vi "APC_9049_FPGA_IGNDI_supervisor.vi"(1 "Time out limit":u32=6000000, 2 "EPTData":T1={"CrankSigOS"=FALSE, "CrankStalled"=FALSE, "SyncStopped"=FALSE, "MissedCrankFlag"=FALSE, "MissedCamFlag"=FALSE, "Period"=588, "PeriodAccum"=3882066, "CrankCount"=5844, "CurrentPosition"=23376, "MAX_CAT"=57600}, 3 "SIarray":bool[](array[boolean])=[FALSE, FALSE, FALSE, FALSE, FALSE, FALSE], 4 "DIarray":bool[](array[boolean])=[FALSE, FALSE, FALSE, FALSE, FALSE, FALSE]) -> (0 "NumberOfActiveIGN_DI":u8)   [LabVIEW 2020]
panel:
  out "Number of inactive injections":u8
  out "Number of inactive sparks":i16
  out "DI6":bool
  out "DI5":bool
  out "DI4":bool
  out "DI3":bool
  out "DI2":bool
  out "DI1":bool
  out "SI6":bool
  out "SI5":bool
  out "SI4":bool
  out "SI3":bool
  out "SI2":bool
  out "SI1":bool
  # "6e6 times out por 800 rpm\n\n2*60/rpm*40e10"
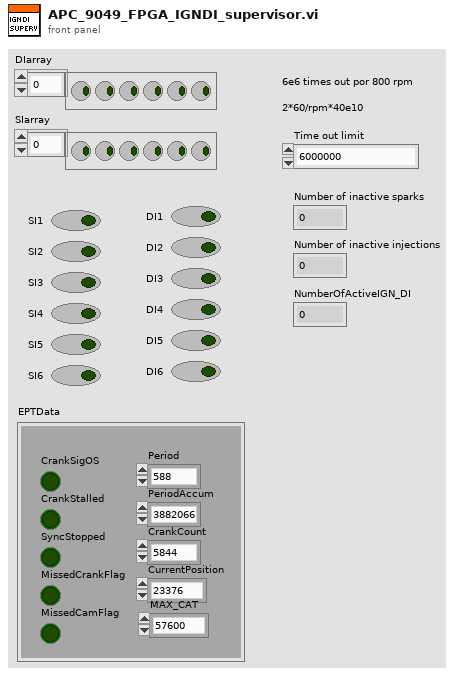
[diagram p1: front panel]
types:
  T1 = cluster{"CrankSigOS":bool, "CrankStalled":bool, "SyncStopped":bool, "MissedCrankFlag":bool, "MissedCamFlag":bool, "Period":u32, "PeriodAccum":u32, "CrankCount":u16, "CurrentPosition":u16, "MAX_CAT":u16}
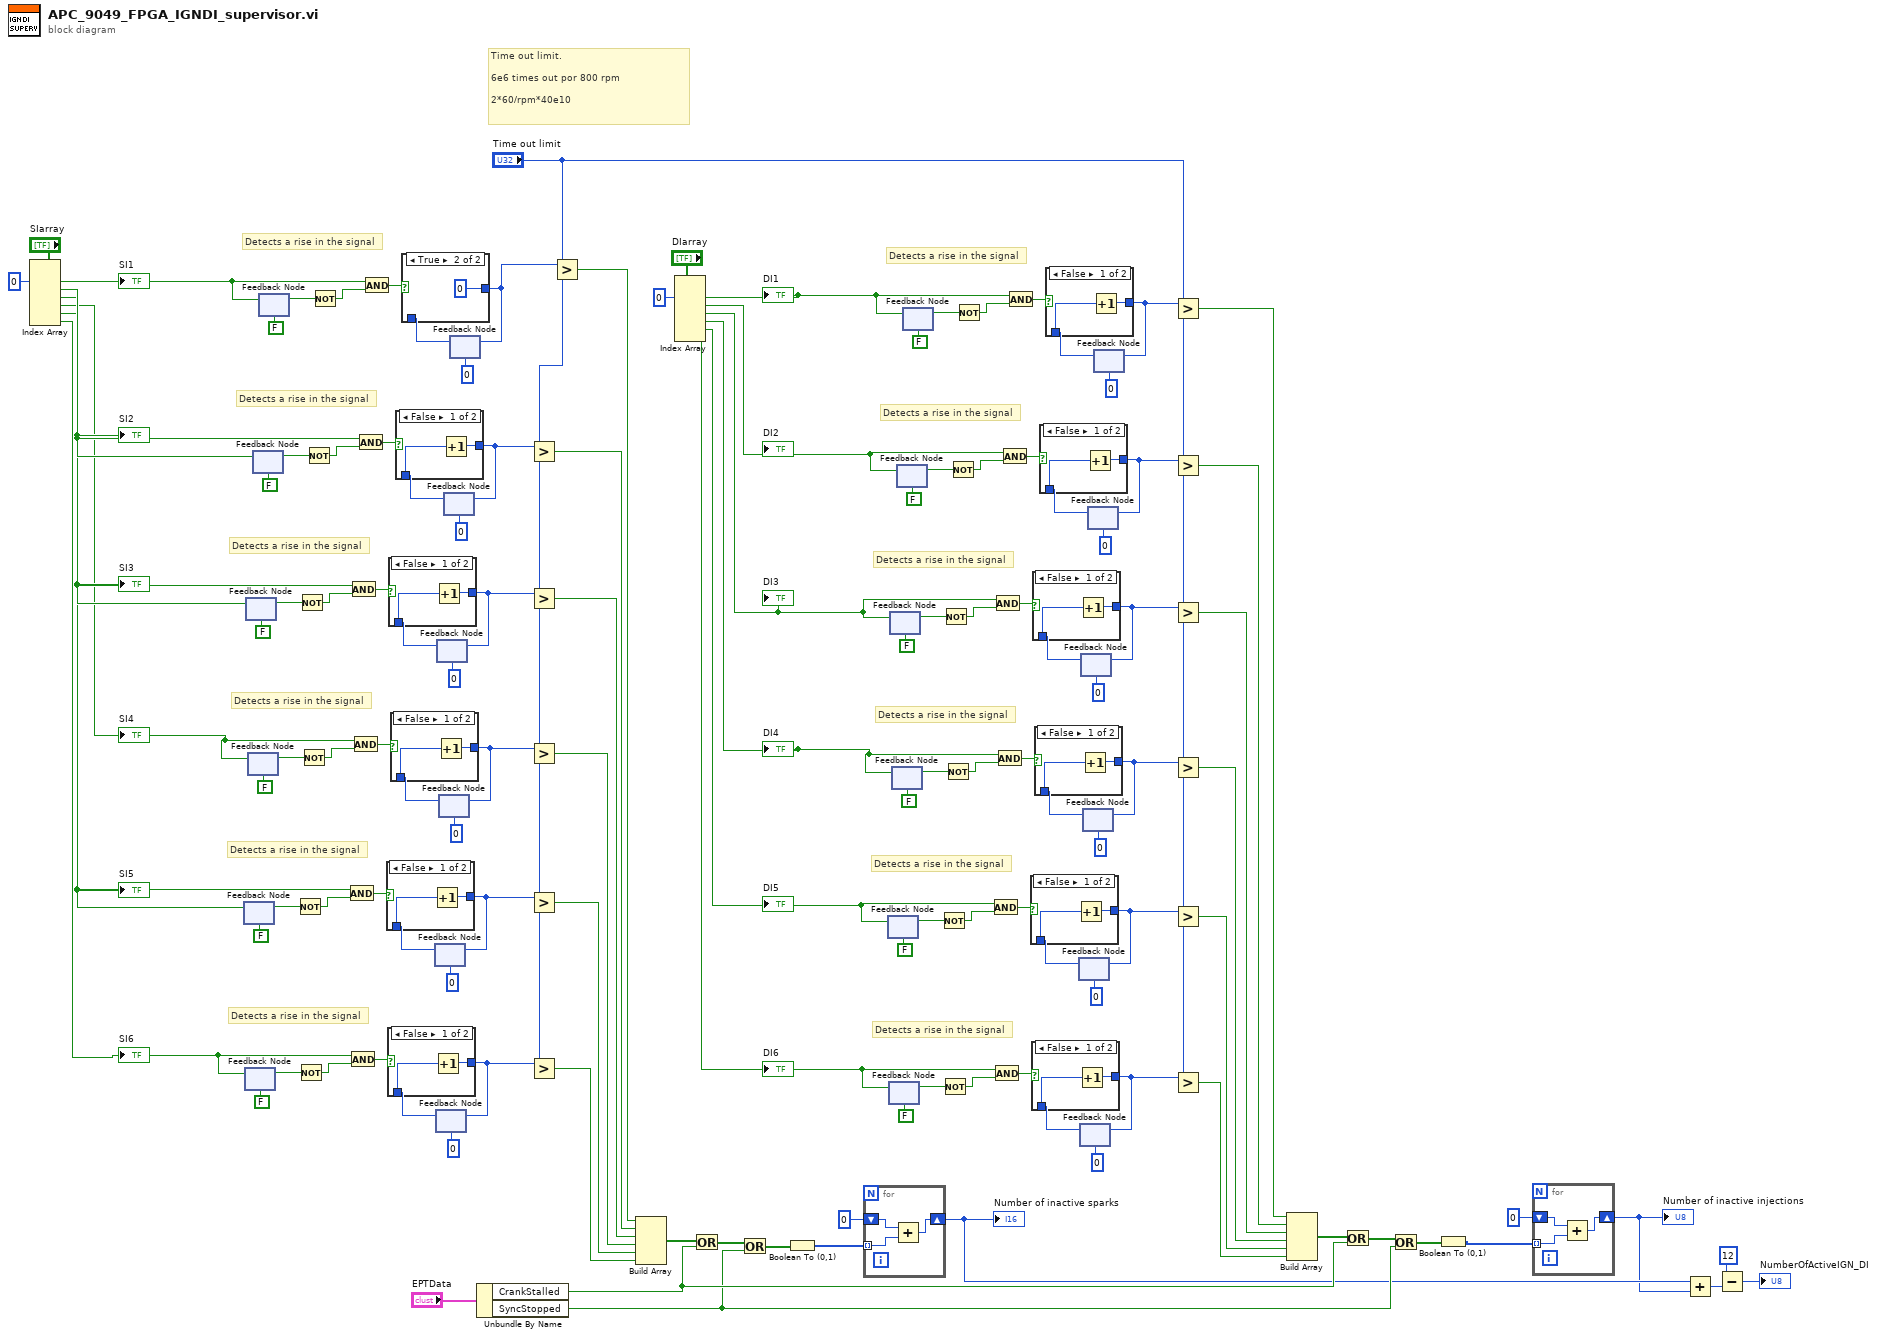
[diagram p0: block diagram]
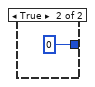
[diagram p2: hidden frame]
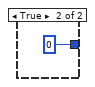
[diagram p3: hidden frame]
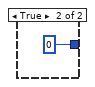
[diagram p4: hidden frame]
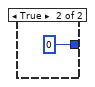
[diagram p5: hidden frame]
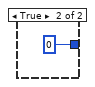
[diagram p6: hidden frame]
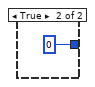
[diagram p7: hidden frame]
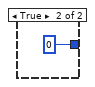
[diagram p8: hidden frame]
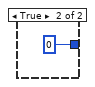
[diagram p9: hidden frame]
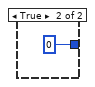
[diagram p10: hidden frame]
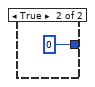
[diagram p11: hidden frame]
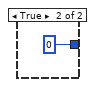
[diagram p12: hidden frame]
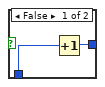
[diagram p13: hidden frame]
diagram:
  # "Detects a rise in the signal"
  # "Detects a rise in the signal"
  # "Detects a rise in the signal"
  # "Detects a rise in the signal"
  # "Detects a rise in the signal"
  # "Detects a rise in the signal"
  # "Detects a rise in the signal"
  # "Detects a rise in the signal"
  # "Detects a rise in the signal"
  # "Detects a rise in the signal"
  # "Detects a rise in the signal"
  # "Time out limit.\n\n6e6 times out por 800 rpm\n\n2*60/rpm*40e10"
  # "Detects a rise in the signal"
  n1 = Index Array(array="SIarray", index #1=0 ("index")) -> (element #1=w6:bool, element #2=w5:bool, element #3=w4:bool, element #4=w3:bool, element #5=w2:bool, element #6=w1:bool)  [unwired: 5 in]
  "SI1" <- w6
  "SI2" <- w5
  "SI3" <- w4
  "SI4" <- w3
  "SI5" <- w2
  "SI6" <- w1
  n2 = feedback #1(FALSE ("x")) -> (w101:bool)
  n3 = feedback-in #1(w2) -> ()
  n4 = feedback #2(FALSE ("x")) -> (w94:bool)
  n5 = feedback-in #2(w1) -> ()
  n6 = feedback #3(FALSE ("x")) -> (w115:bool)
  n7 = feedback-in #3(w4) -> ()
  n8 = feedback #4(FALSE ("x")) -> (w108:bool)
  n9 = feedback-in #4(w3) -> ()
  n10 = feedback #5(FALSE ("x")) -> (w122:bool)
  n11 = feedback-in #5(w5) -> ()
  n12 = feedback-in #6(w6) -> ()
  n13 = feedback #6(FALSE ("x")) -> (w130:bool)
  n14 = Not(x=w101) -> (.not. x?=w102:bool)
  n15 = Not(x=w94) -> (.not. x?=w95:bool)
  n16 = Not(x=w115) -> (.not. x?=w116:bool)
  n17 = Not(x=w108) -> (.not. x?=w109:bool)
  n18 = Not(x=w122) -> (.not. x?=w123:bool)
  n19 = Not(x=w130) -> (.not. x?=w131:bool)
  n20 = And(x=w2, y=w102) -> (x .and. y?=w99:bool)
  n21 = And(x=w1, y=w95) -> (x .and. y?=w92:bool)
  n22 = And(x=w4, y=w116) -> (x .and. y?=w113:bool)
  n23 = And(x=w3, y=w109) -> (x .and. y?=w106:bool)
  n24 = And(x=w5, y=w123) -> (x .and. y?=w120:bool)
  n25 = And(x=w6, y=w131) -> (x .and. y?=w128:bool)
  n26 = feedback #7(u32 0) -> (w98:u32)
  n27 = case shown="False" w99 {
    tunnel: [w133 u32 0] -> w96
    tunnel: w98 -> [w132 _]
    frame False {
      n28 = Increment(x=w132) -> (x+1=w133:u32)
    }
    frame True {
    }
  }
  n29 = feedback-in #7(w96) -> ()
  n30 = feedback #8(u32 0) -> (w91:u32)
  n31 = case shown="False" w92 {
    tunnel: [w136 u32 0] -> w89
    tunnel: w91 -> [w135 _]
    frame False {
      n32 = Increment(x=w135) -> (x+1=w136:u32)
    }
    frame True {
    }
  }
  n33 = feedback-in #8(w89) -> ()
  n34 = feedback #9(u32 0) -> (w112:u32)
  n35 = case shown="False" w113 {
    tunnel: [w139 u32 0] -> w110
    tunnel: w112 -> [w138 _]
    frame False {
      n36 = Increment(x=w138) -> (x+1=w139:u32)
    }
    frame True {
    }
  }
  n37 = feedback-in #9(w110) -> ()
  n38 = feedback #10(u32 0) -> (w105:u32)
  n39 = case shown="False" w106 {
    tunnel: [w142 u32 0] -> w103
    tunnel: w105 -> [w141 _]
    frame False {
      n40 = Increment(x=w141) -> (x+1=w142:u32)
    }
    frame True {
    }
  }
  n41 = feedback-in #10(w103) -> ()
  n42 = feedback #11(u32 0) -> (w119:u32)
  n43 = case shown="False" w120 {
    tunnel: [w145 u32 0] -> w117
    tunnel: w119 -> [w144 _]
    frame False {
      n44 = Increment(x=w144) -> (x+1=w145:u32)
    }
    frame True {
    }
  }
  n45 = feedback-in #11(w117) -> ()
  n46 = feedback #12(u32 0) -> (w127:u32)
  n47 = case shown="True" w128 {
    tunnel: [w148 u32 0] -> w125
    tunnel: w127 -> [w147 _]
    frame False {
      n48 = Increment(x=w147) -> (x+1=w148:u32)
    }
    frame True {
    }
  }
  n49 = feedback-in #12(w125) -> ()
  n50 = Unbundle By Name("EPTData") -> ("CrankStalled"=w33:bool, "SyncStopped"=w32:bool)
  n51 = Greater?(x=w117, y="Time out limit") -> (0:w44:bool)
  n52 = Greater?(x=w110, y="Time out limit") -> (0:w43:bool)
  n53 = Greater?(x=w103, y="Time out limit") -> (0:w42:bool)
  n54 = Greater?(x=w96, y="Time out limit") -> (0:w41:bool)
  n55 = Greater?(x=w89, y="Time out limit") -> (0:w40:bool)
  n56 = Greater?(x=w125, y="Time out limit") -> (0:w45:bool)
  n57 = Build Array(w45, w44, w43, w42, w41, w40) -> (w39:bool[])
  n58 = Index Array(array="DIarray", index #1=0 ("index")) -> (element #1=w14:bool, element #2=w13:bool, element #3=w12:bool, element #4=w11:bool, element #5=w10:bool, element #6=w9:bool)  [unwired: 5 in]
  "DI1" <- w14
  "DI2" <- w13
  "DI3" <- w12
  "DI4" <- w11
  "DI5" <- w10
  "DI6" <- w9
  n59 = Or(x=w39, y=w33) -> (x .or. y?=w38:bool[])
  n60 = Or(x=w38, y=w32) -> (x .or. y?=w37:bool[])
  n61 = Boolean To (0,1)(Boolean=w37) -> (0, 1=w24:i16[])
  n62 = for {
    shift-right: [w152] -> w21
    shift-left: i16 0 -> [w151]
    tunnel: w24 -> [w150] mode=indexing
    n63 = Add(x=w151, y=w150) -> (x+y=w152:i16)
  }
  "Number of inactive sparks" <- w21
  n64 = feedback #13(FALSE ("x")) -> (w59:bool)
  n65 = feedback-in #13(w10) -> ()
  n66 = feedback #14(FALSE ("x")) -> (w52:bool)
  n67 = feedback-in #14(w9) -> ()
  n68 = feedback #15(FALSE ("x")) -> (w73:bool)
  n69 = feedback-in #15(w12) -> ()
  n70 = feedback #16(FALSE ("x")) -> (w66:bool)
  n71 = feedback-in #16(w11) -> ()
  n72 = feedback #17(FALSE ("x")) -> (w80:bool)
  n73 = feedback-in #17(w13) -> ()
  n74 = feedback #18(FALSE ("x")) -> (w87:bool)
  n75 = feedback-in #18(w14) -> ()
  n76 = Not(x=w59) -> (.not. x?=w60:bool)
  n77 = Not(x=w52) -> (.not. x?=w53:bool)
  n78 = Not(x=w73) -> (.not. x?=w74:bool)
  n79 = Not(x=w66) -> (.not. x?=w67:bool)
  n80 = Not(x=w80) -> (.not. x?=w81:bool)
  n81 = Not(x=w87) -> (.not. x?=w88:bool)
  n82 = And(x=w10, y=w60) -> (x .and. y?=w57:bool)
  n83 = And(x=w9, y=w53) -> (x .and. y?=w50:bool)
  n84 = And(x=w12, y=w74) -> (x .and. y?=w71:bool)
  n85 = And(x=w11, y=w67) -> (x .and. y?=w64:bool)
  n86 = And(x=w13, y=w81) -> (x .and. y?=w78:bool)
  n87 = And(x=w14, y=w88) -> (x .and. y?=w85:bool)
  n88 = feedback #19(u32 0) -> (w56:u32)
  n89 = case shown="False" w57 {
    tunnel: [w154 u32 0] -> w54
    tunnel: w56 -> [w153 _]
    frame False {
      n90 = Increment(x=w153) -> (x+1=w154:u32)
    }
    frame True {
    }
  }
  n91 = feedback-in #19(w54) -> ()
  n92 = feedback #20(u32 0) -> (w49:u32)
  n93 = case shown="False" w50 {
    tunnel: [w157 u32 0] -> w47
    tunnel: w49 -> [w156 _]
    frame False {
      n94 = Increment(x=w156) -> (x+1=w157:u32)
    }
    frame True {
    }
  }
  n95 = feedback-in #20(w47) -> ()
  n96 = feedback #21(u32 0) -> (w70:u32)
  n97 = case shown="False" w71 {
    tunnel: [w160 u32 0] -> w68
    tunnel: w70 -> [w159 _]
    frame False {
      n98 = Increment(x=w159) -> (x+1=w160:u32)
    }
    frame True {
    }
  }
  n99 = feedback-in #21(w68) -> ()
  n100 = feedback #22(u32 0) -> (w63:u32)
  n101 = case shown="False" w64 {
    tunnel: [w163 u32 0] -> w61
    tunnel: w63 -> [w162 _]
    frame False {
      n102 = Increment(x=w162) -> (x+1=w163:u32)
    }
    frame True {
    }
  }
  n103 = feedback-in #22(w61) -> ()
  n104 = feedback #23(u32 0) -> (w77:u32)
  n105 = case shown="False" w78 {
    tunnel: [w166 u32 0] -> w75
    tunnel: w77 -> [w165 _]
    frame False {
      n106 = Increment(x=w165) -> (x+1=w166:u32)
    }
    frame True {
    }
  }
  n107 = feedback-in #23(w75) -> ()
  n108 = feedback #24(u32 0) -> (w84:u32)
  n109 = case shown="False" w85 {
    tunnel: [w169 u32 0] -> w82
    tunnel: w84 -> [w168 _]
    frame False {
      n110 = Increment(x=w168) -> (x+1=w169:u32)
    }
    frame True {
    }
  }
  n111 = feedback-in #24(w82) -> ()
  n112 = Greater?(x=w82, y="Time out limit") -> (0:w31:bool)
  n113 = Greater?(x=w75, y="Time out limit") -> (0:w30:bool)
  n114 = Greater?(x=w68, y="Time out limit") -> (0:w29:bool)
  n115 = Greater?(x=w61, y="Time out limit") -> (0:w28:bool)
  n116 = Greater?(x=w54, y="Time out limit") -> (0:w27:bool)
  n117 = Greater?(x=w47, y="Time out limit") -> (0:w26:bool)
  n118 = Build Array(w31, w30, w29, w28, w27, w26) -> (w36:bool[])
  n119 = Or(x=w36, y=w33) -> (x .or. y?=w35:bool[])
  n120 = Or(x=w35, y=w32) -> (x .or. y?=w34:bool[])
  n121 = Boolean To (0,1)(Boolean=w34) -> (0, 1=w22:i16[])
  n122 = for {
    shift-right: [w173] -> w20
    shift-left: u8 0 -> [w172]
    tunnel: w22 -> [w171] mode=indexing
    n123 = Add(x=w172, y=w171) -> (x+y=w173:i16)
  }
  "Number of inactive injections" <- w20
  n124 = Add(x=w21, y=w20) -> (x+y=w19:i16)
  n125 = Subtract(x=u8 12, y=w19) -> (x-y=→"NumberOfActiveIGN_DI":i16)
